vi "顺序结构.vi"() -> ()   [LabVIEW 2019]
panel:
  out "x-y 4":u32
  out "x-y 3":u32
  out "x-y 2":u32
  out "x-y":u32
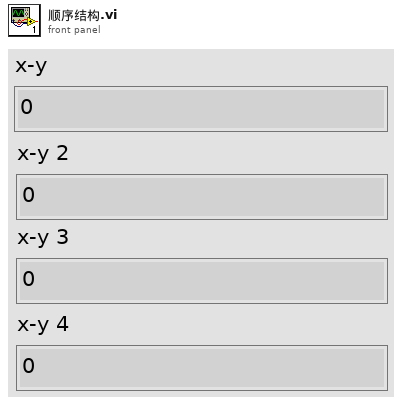
[diagram p1: front panel]
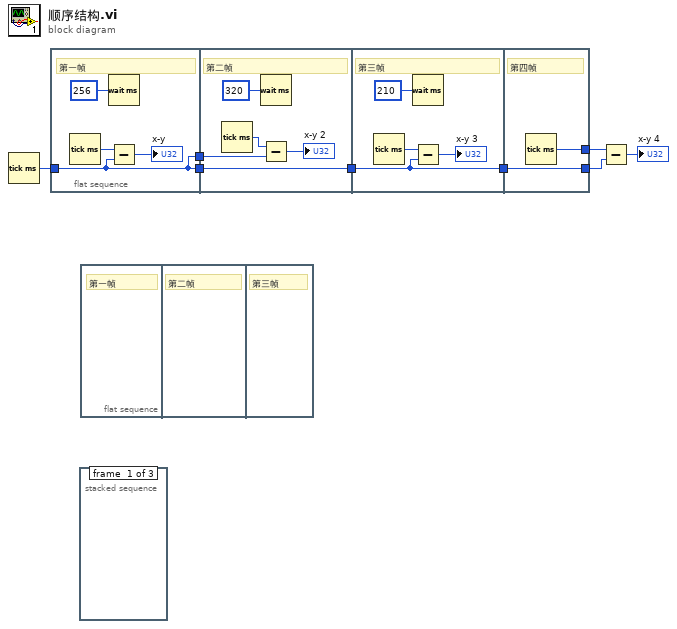
[diagram p0: block diagram]
diagram:
  n1 = Tick Count (ms)() -> (millisecond timer value=w8:u32)
  n2 = flat-sequence {
    tunnel: w8 -> [w9]
    tunnel: [w9] -> w7
    tunnel: [w9] -> w5
    tunnel: w7 -> [w15]
    tunnel: [w13] -> w6
    tunnel: w5 -> [w13]
    tunnel: w6 -> [w18]
    tunnel: [w18] -> w3
    tunnel: [w23] -> w1
    tunnel: w3 -> [w23]
    tunnel: [w22] -> w2
    frame #0 {
      # "第一帧"
      n3 = Tick Count (ms)() -> (millisecond timer value=w12:u32)
      n4 = Wait (ms)(milliseconds to wait=u32 256 ("等待时间（毫秒）")) -> ()  [unwired: 1 out]
      n5 = Subtract(x=w12, y=w9) -> (x-y=→"x-y":u32)
    }
    frame #1 {
      # "第二帧"
      n6 = Tick Count (ms)() -> (millisecond timer value=w16:u32)
      n7 = Wait (ms)(milliseconds to wait=u32 320 ("等待时间（毫秒）")) -> ()  [unwired: 1 out]
      n8 = Subtract(x=w16, y=w15) -> (x-y=→"x-y 2":u32)
    }
    frame #2 {
      # "第三帧"
      n9 = Tick Count (ms)() -> (millisecond timer value=w20:u32)
      n10 = Wait (ms)(milliseconds to wait=u32 210 ("等待时间（毫秒）")) -> ()  [unwired: 1 out]
      n11 = Subtract(x=w20, y=w18) -> (x-y=→"x-y 3":u32)
    }
    frame #3 {
      # "第四帧"
      n12 = Tick Count (ms)() -> (millisecond timer value=w22:u32)
    }
  }
  n13 = stacked-sequence {
    frame #0 {
    }
    frame #1 {
    }
    frame #2 {
    }
  }
  n14 = flat-sequence {
    frame #0 {
      # "第一帧"
    }
    frame #1 {
      # "第二帧"
    }
    frame #2 {
      # "第三帧"
    }
  }
  n15 = Subtract(x=w2, y=w1) -> (x-y=→"x-y 4":u32)
